vi "ReadConfig.vi"(8 "error in (no error)":errorcluster, 11 "RoomAlert in":refnum<class "RoomAlert.lvclass">) -> (0 "error out":errorcluster, 2 "Config":variant, 3 "RoomAlert out":refnum<class "RoomAlert.lvclass">)   [LabVIEW 2018, in "SensorPlugins.lvlib" / "RoomAlert.lvclass"]
uses:
  RoomAlert.lvclass
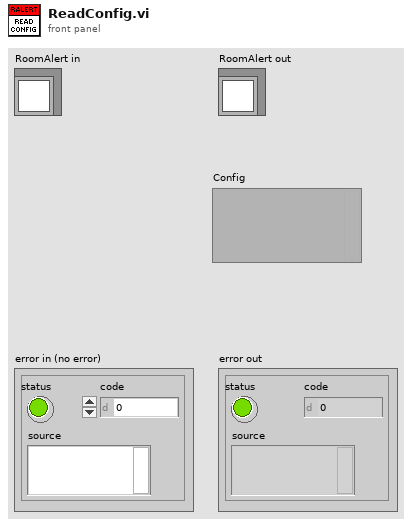
[diagram p1: front panel]
types:
  T1 = typedef "SensorPlugins.lvlib/RoomAlert.lvclass/RoomAlertControls.ctl" = cluster{"Connected?":bool, "IP Address of SNMP Device":string, "Port (502)":u16, "GET OID ARRAY":string[], "SET OID ARRAY":string[][], "Community Name":string, "Measurements To Read Array":u16[], "Use Measurement To Read Array":bool}[]
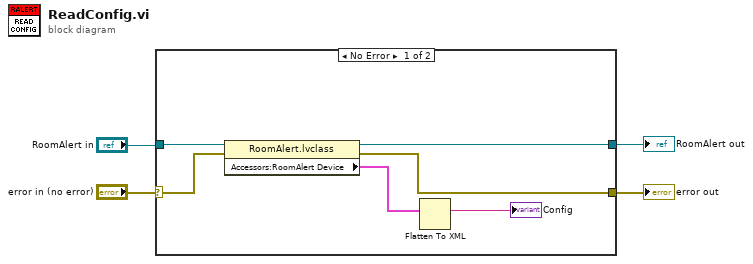
[diagram p0: block diagram]
diagram:
  n1 = case shown="No Error" "error in (no error)" {
    selector: "error in (no error)" -> [w8 w12]
    tunnel: "RoomAlert in" -> [w10 w11]
    tunnel: [w7 w12] -> w1
    tunnel: [w9 w11] -> w2
    frame No Error {
      n2 = property class="RoomAlert.lvclass"(reference=w10, error in=w8) -> (reference out=w9:refnum<class "RoomAlert.lvclass">, error out=w7:errorcluster, "Accessors:RoomAlert Device"=w6:T1)
      n3 = Flatten To XML(anything=w6) -> (xml string=→"Config":string)
    }
    frame Error {
    }
  }
  "error out" <- w1
  "RoomAlert out" <- w2
